vi "Begin[Conflict 1].vi"() -> (0 "Joystick 1 Error":errorcluster)   [LabVIEW 2013]
doc: "Called before other user functions, this VI is expected to open initial I/O refnums, load in file data, and do all program initialization. Notice that the <B>error out</B> terminal is simply used for data flow. Wiring it to other structures or subVIs ensures that this VI runs first."
uses:
  <vilib>/Rock Robotics/SystemInterfaces/DIO/FPGA_DIOPWMChannel.ctl
  <vilib>/Rock Robotics/WPI/SafetyOutput/WPI_SafetyOutputConfigMenu.ctl
  <vilib>/Rock Robotics/WPI/DriverStation/WPI_DriverStationRobotMode2.ctl
  <vilib>/Rock Robotics/SystemInterfaces/Typedef/FPGA_TypedefAnalogModuleForGyro.ctl
  <vilib>/Rock Robotics/SystemInterfaces/AI/FPGA_AIGyroChannel.ctl
  <vilib>/Rock Robotics/WPI/Joystick/WPI_JoystickDeviceEnum.ctl
  <vilib>/Rock Robotics/SystemInterfaces/DIO/FPGA_DIOChannel.ctl
  <vilib>/Rock Robotics/SystemInterfaces/DIO/FPGA_DIORelayChannel.ctl
  <vilib>/Rock Robotics/SystemInterfaces/Typedef/FPGA_TypedefSolenoidModule.ctl
  <vilib>/Rock Robotics/WPI/Solenoid/WPI_SolenoidChannel.ctl
  <vilib>/Rock Robotics/WPI/Solenoid/WPI_SolenoidValue.ctl
  <vilib>/Rock Robotics/WPI/RobotDrive/WPI_RobotDriveOpen2MotorWithTalon.vi
  Robot Global Data.vi
  <vilib>/Rock Robotics/WPI/Solenoid/WPI_SolenoidOpenDouble.vi
  <vilib>/Rock Robotics/WPI/Solenoid/WPI_SolenoidSetEnum.vi
  <vilib>/Rock Robotics/WPI/Solenoid/WPI_SolenoidOpenSingle.vi
  <vilib>/Rock Robotics/WPI/Compressor/WPI_CompressorGetSetRefNum.vi
panel:
  out "Motor Error":errorcluster
  out "Joystick 3 Error":errorcluster
  out "Gyro Open Error":errorcluster
  out "Joystick 2 Error":errorcluster
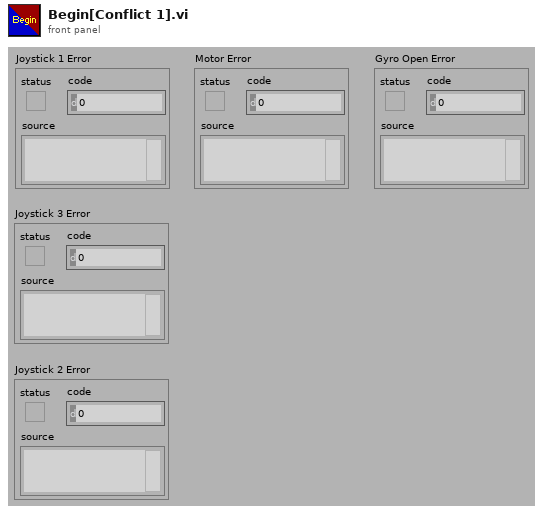
[diagram p1: front panel]
types:
  T1 = typedef "FPGA_DIORelayChannel.ctl" = enum8{"Relay 1", "Relay 2", "Relay 3", "Relay 4", "Relay 5", "Relay 6", "Relay 7", "Relay 8", "Invalid"}
  T2 = typedef "FPGA_DIOChannel.ctl" = enum8{"DIO 1", "DIO 2", "DIO 3", "DIO 4", "DIO 5", "DIO 6", "DIO 7", "DIO 8", "DIO 9", "DIO 10", "DIO 11", "DIO 12", "DIO 13", "DIO 14", "Invalid"}
  T3 = typedef "WPI_JoystickDeviceEnum.ctl" = enum16{"USB 1", "USB 2", "USB 3", "USB 4", "Kinect 1", "Kinect 2"}
  T4 = typedef "FPGA_AIGyroChannel.ctl" = enum8{"AI 1", "AI 2", "Invalid"}
  T5 = typedef "FPGA_TypedefAnalogModuleForGyro.ctl" = enum16{"Analog Module 1"}
  T6 = typedef "WPI_DriverStationRobotMode2.ctl" = enum16{"Autonomous Disabled", "Autonomous Enabled", "Teleop Disabled", "Teleop Enabled", "Timeout", "Finish", "Test Disabled", "Test Enabled"}
  T7 = typedef "WPI_SafetyOutputConfigMenu.ctl" = enum16{"Enable", "Disable"}
  T8 = typedef "FPGA_DIOPWMChannel.ctl" = enum8{"PWM 1", "PWM 2", "PWM 3", "PWM 4", "PWM 5", "PWM 6", "PWM 7", "PWM 8", "PWM 9", "PWM 10", "Invalid"}
  T9 = typedef "WPI_SolenoidChannel.ctl" = enum8{"Solenoid 1", "Solenoid 2", "Solenoid 3", "Solenoid 4", "Solenoid 5", "Solenoid 6", "Solenoid 7", "Solenoid 8", "Invalid"}
  T10 = typedef "FPGA_TypedefSolenoidModule.ctl" = enum16{"Solenoid Module 1", "Solenoid Module 2"}
  T11 = typedef "WPI_SolenoidDevRef.ctl" = cluster{"DevStatus":errorcluster, "Solenoid Module":T10, "Forward Solenoid Channel":T9, "Reverse Solenoid Channel":T9}
  T12 = typedef "WPI_SolenoidValue.ctl" = enum16{"Off", "On", "Forward", "Reverse"}
  T13 = typedef "WPI_JoystickDevRef.ctl" = cluster{"Device":T3}
  T14 = typedef "WPI_CompressorDevRef.ctl" = cluster{"DevStatus":errorcluster, "DigitalInputDevRef":T15, "RelayDevRef":T17}
  T15 = typedef "WPI_DigitalInputDevRef.ctl" = cluster{"DevStatus":errorcluster, "DIO Channel":T2, "Digital Module":T16}
  T16 = typedef "FPGA_TypedefDigitalModule.ctl" = enum16{"Digital Module 1", "Digital Module 2"}
  T17 = typedef "WPI_RelayDevRef.ctl" = cluster{"DevStatus":errorcluster, "Relay Channel":T1, "Digital Module":T16, "Relay Direction":T18}
  T18 = typedef "WPI_RelayDirection.ctl" = enum16{"Both directions", "Forward only", "Reverse only"}
  T19 = typedef "WPI_GyroDevRef.ctl" = cluster{"DevStatus":errorcluster, "Analog Module":T20, "Analog Channel":T21, "Offset":dbl, "Gain (VoltsPerDegree/Second)":dbl}
  T20 = typedef "FPGA_TypedefAnalogModule.ctl" = enum16{"Analog Module 1", "Analog Module 2"}
  T21 = typedef "FPGA_AIChannel.ctl" = enum8{"AI 1", "AI 2", "AI 3", "AI 4", "AI 5", "AI 6", "AI 7", "AI 8", "Invalid"}
  T22 = typedef "WPI_RobotDriveDevRef.ctl" = cluster{"DevStatus":errorcluster, "Motors[]":T23[], "Square Inputs":bool, "Max Output":dbl, "Isochronous":bool}
  T23 = typedef "WPI_MotorControlDeviceRef.ctl" = cluster{"DeviceStatus":errorcluster, "Type":enum16{"PWM", "CAN"}, "PWM":cluster{"Digital Module":T16, "PWM Channel":T8, "DeadBand":T24}, "CAN":cluster{"Device Number":u8, "Control Mode":T25, "Semaphore":T26, "Max Vout":dbl}, "Invert":bool, "TransformRef":T27, "InvTransformRef":T27}
  T24 = typedef "WPI_PWMDeadband.ctl" = cluster{"Name":string, "maxPositivePwm":i32, "minPositivePwm":i32, "centerPwm":i32, "maxNegativePwm":i32, "minNegativePwm":i32, "angularRange":u16}
  T25 = typedef "WPI_CANJaguar_ControlMode.ctl" = enum8{"Percent VBus", "Current", "Speed", "Position", "Voltage"}
  T26 = typedef "Semaphore RefNum" = refnum<k1>
  T27 = typedef "WPI_PWMTransform_ConPane.ctl" = refnum<vi>
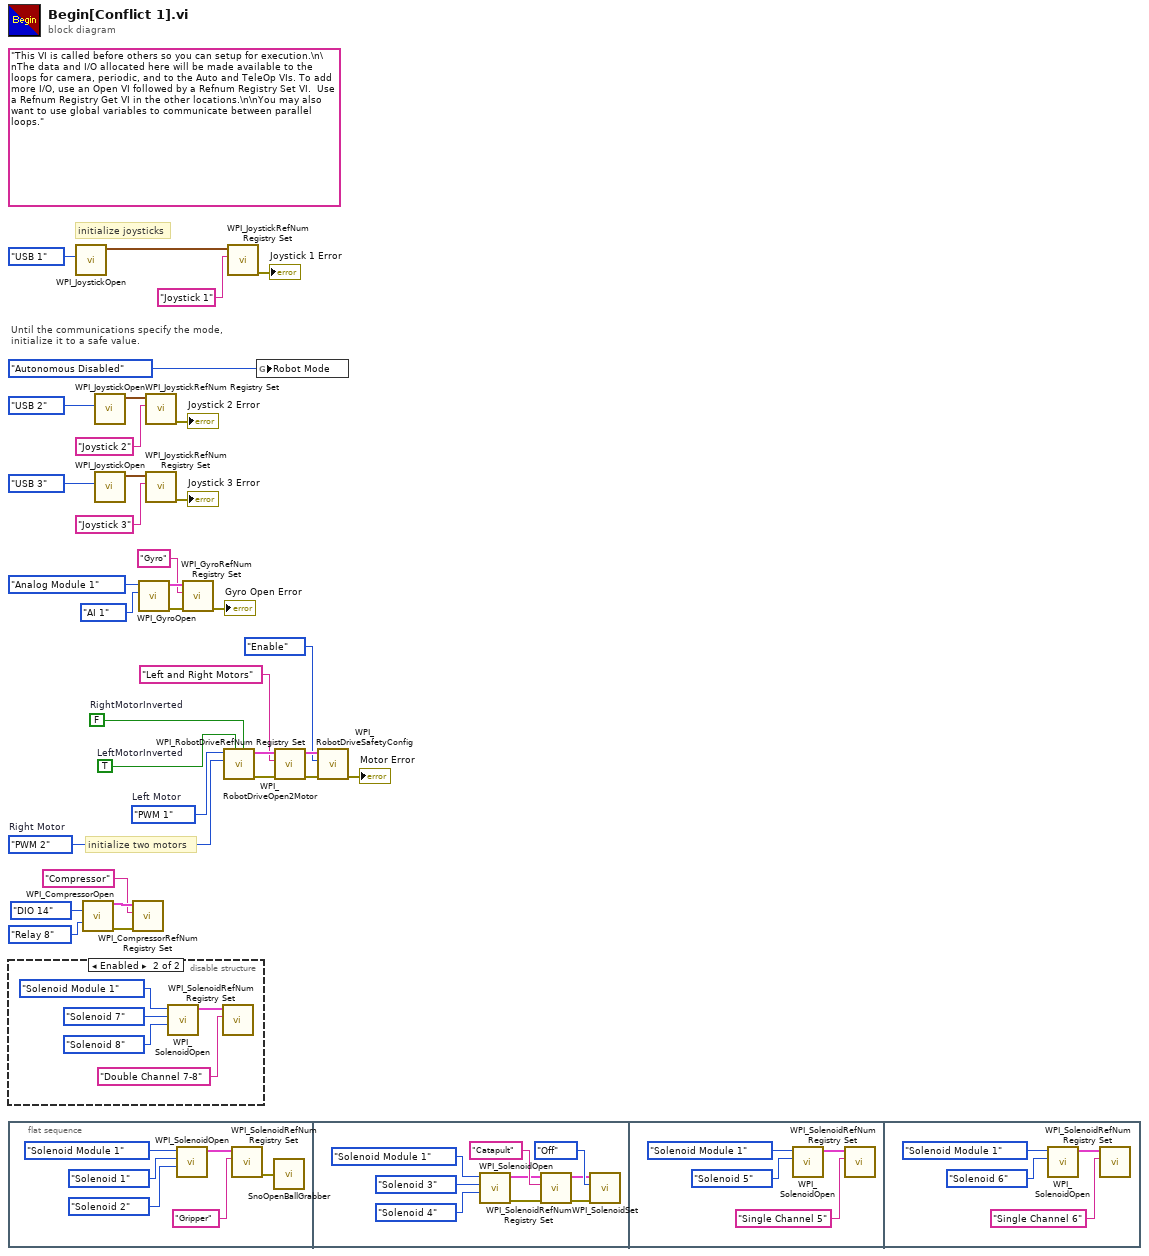
[diagram p0: block diagram]
diagram:
  (unwired) "This VI is called before others so you can setup for execution.\n\nThe data and I/O allocated here will be made available to the loops for camera, periodic, and to the Auto and TeleOp VIs. To add more I/O, use an Open VI followed by a Refnum Registry Set VI.  Use a Refnum Registry Get VI in the other locations.\n\nYou may also want to use global variables to communicate between parallel loops."
  w29 = FPGA_DIOPWMChannel."PWM 2"  # Right Motor
  w30 = FPGA_DIOPWMChannel."PWM 1"  # Left Motor
  w34 = TRUE  # LeftMotorInverted
  w35 = FALSE  # RightMotorInverted
  # "initialize joysticks"
  # "Until the communications specify the mode,\ninitialize it to a safe value."
  # "initialize two motors"
  n1 = disable-structure shown="Enabled" {
    frame Disabled {
    }
    frame Enabled {
      n2 = call-poly <vilib>:"WPI_SolenoidOpen.vi"("Reverse Solenoid Channel"=WPI_SolenoidChannel."Solenoid 8", "Forward Solenoid Channel"=WPI_SolenoidChannel."Solenoid 7", "Solenoid Module (Module 1)"=FPGA_TypedefSolenoidModule."Solenoid Module 1") -> ("SolenoidDevRef"=w39:T11)  [unwired: 7 in, 1 out]
      n3 = call <vilib>:"WPI_SolenoidRefNum Registry Set.vi"("refnum name"="Double Channel 7-8", "SolenoidDevRef"=w39) -> ()  [unwired: 8 in, 2 out]
    }
  }
  n4 = flat-sequence {
    frame #0 {
      n5 = call-poly <vilib>:"WPI_SolenoidOpen.vi"("Reverse Solenoid Channel"=WPI_SolenoidChannel."Solenoid 2", "Forward Solenoid Channel"=WPI_SolenoidChannel."Solenoid 1", "Solenoid Module (Module 1)"=FPGA_TypedefSolenoidModule."Solenoid Module 1") -> ("SolenoidDevRef"=w46:T11)  [unwired: 7 in, 1 out]
      n6 = call <vilib>:"WPI_SolenoidRefNum Registry Set.vi"("refnum name"="Gripper", "SolenoidDevRef"=w46) -> ("error out"=w41:errorcluster)  [unwired: 8 in, 1 out]
      n7 = call "SnoOpenBallGrabber.vi"("Input Error"=w41) -> ()  [unwired: 1 out]
    }
    frame #1 {
      n8 = call-poly <vilib>:"WPI_SolenoidOpen.vi"("Reverse Solenoid Channel"=WPI_SolenoidChannel."Solenoid 4", "Forward Solenoid Channel"=WPI_SolenoidChannel."Solenoid 3", "Solenoid Module (Module 1)"=FPGA_TypedefSolenoidModule."Solenoid Module 1") -> ("error out"=w51:errorcluster, "SolenoidDevRef"=w50:T11)  [unwired: 7 in]
      n9 = call <vilib>:"WPI_SolenoidRefNum Registry Set.vi"("error in (no error)"=w51, "refnum name"="Catapult", "SolenoidDevRef"=w50) -> ("error out"=w54:errorcluster, "SolenoidDevRef"=w53:T11)  [unwired: 7 in]
      n10 = call-poly <vilib>:"WPI_SolenoidSet.vi"("error in (no error)"=w54, "Value"=WPI_SolenoidValue."Off", "SolenoidDevRef"=w53) -> ()  [unwired: 7 in, 2 out]
    }
    frame #2 {
      n11 = call-poly <vilib>:"WPI_SolenoidOpen.vi"("Solenoid Channel"=WPI_SolenoidChannel."Solenoid 5" ("Forward Solenoid Channel"), "Solenoid Module (Module 1)"=FPGA_TypedefSolenoidModule."Solenoid Module 1") -> ("SolenoidDevRef"=w58:T11)  [unwired: 8 in, 1 out]
      n12 = call <vilib>:"WPI_SolenoidRefNum Registry Set.vi"("refnum name"="Single Channel 5", "SolenoidDevRef"=w58) -> ()  [unwired: 8 in, 2 out]
    }
    frame #3 {
      n13 = call-poly <vilib>:"WPI_SolenoidOpen.vi"("Solenoid Channel"=WPI_SolenoidChannel."Solenoid 6" ("Forward Solenoid Channel"), "Solenoid Module (Module 1)"=FPGA_TypedefSolenoidModule."Solenoid Module 1") -> ("SolenoidDevRef"=w62:T11)  [unwired: 8 in, 1 out]
      n14 = call <vilib>:"WPI_SolenoidRefNum Registry Set.vi"("refnum name"="Single Channel 6", "SolenoidDevRef"=w62) -> ()  [unwired: 8 in, 2 out]
    }
  }
  n15 = call <vilib>:"WPI_JoystickOpen.vi"("JoystickDevice"=WPI_JoystickDeviceEnum."USB 1") -> ("JoystickDevRef"=w13:T13)  [unwired: 10 in]
  n16 = call <vilib>:"WPI_CompressorOpen.vi"("Pressure Switch DIO Channel"=FPGA_DIOChannel."DIO 14", "Relay Channel"=FPGA_DIORelayChannel."Relay 8") -> ("CompressorDevRef"=w3:T14, "error out"=w2:errorcluster)  [unwired: 12 in]
  n17 = call <vilib>:"WPI_JoystickOpen.vi"("JoystickDevice"=WPI_JoystickDeviceEnum."USB 2") -> ("JoystickDevRef"=w17:T13)  [unwired: 10 in]
  n18 = call <vilib>:"WPI_JoystickOpen.vi"("JoystickDevice"=WPI_JoystickDeviceEnum."USB 3") -> ("JoystickDevRef"=w9:T13)  [unwired: 10 in]
  n19 = call <vilib>:"WPI_CompressorRefNum Registry Set.vi"("error in (no error)"=w2, "refnum name"="Compressor", "CompressorDevRef"=w3) -> ()  [unwired: 7 in, 2 out]
  n20 = call <vilib>:"WPI_GyroOpen.vi"("Analog Channel"=FPGA_AIGyroChannel."AI 1", "Analog Module (Module 1)"=FPGA_TypedefAnalogModuleForGyro."Analog Module 1") -> ("error out"=w21:errorcluster, "GyroDevRef"=w23:T19)  [unwired: 7 in, 1 out]
  n21 = call <vilib>:"WPI_JoystickRefNum Registry Set.vi"("refnum name"="Joystick 2", "JoystickDevRef"=w17) -> ("error out"=→"Joystick 2 Error":errorcluster)  [unwired: 8 in, 1 out]
  n22 = call <vilib>:"WPI_JoystickRefNum Registry Set.vi"("refnum name"="Joystick 3", "JoystickDevRef"=w9) -> ("error out"=→"Joystick 3 Error":errorcluster)  [unwired: 8 in, 1 out]
  n23 = call <vilib>:"WPI_GyroRefNum Registry Set.vi"("error in (no error)"=w21, "refnum name"="Gyro", "GyroDevRef"=w23) -> ("error out"=→"Gyro Open Error":errorcluster)  [unwired: 7 in, 1 out]
  n24 = call-poly <vilib>:"WPI_RobotDriveOpen2Motor.vi"("Right Motor Inverted"=w35, "Left Motor Inverted"=w34, "Right Motor"=w29, "Left Motor"=w30) -> ("error out"=w31:errorcluster, "RobotDriveDevRef"=w33:T22)  [unwired: 1 in, 5 out]
  n25 = call <vilib>:"WPI_JoystickRefNum Registry Set.vi"("refnum name"="Joystick 1", "JoystickDevRef"=w13) -> ("error out"=→"Joystick 1 Error":errorcluster)  [unwired: 8 in, 1 out]
  n26 = global write "Robot Global Data.vi" "Robot Mode"(WPI_DriverStationRobotMode2."Autonomous Disabled" ("Robot Mode")) -> ()
  n27 = call <vilib>:"WPI_RobotDriveRefNum Registry Set.vi"("error in (no error)"=w31, "refnum name"="Left and Right Motors", "RobotDriveDevRef"=w33) -> ("error out"=w7:errorcluster, "RobotDriveDevRef"=w28:T22)  [unwired: 7 out]
  n28 = call <vilib>:"WPI_RobotDriveSafetyConfig.vi"("error in (no error)"=w7, "mode"=WPI_SafetyOutputConfigMenu."Enable", "RobotDriveDevRef"=w28) -> ("error out"=→"Motor Error":errorcluster)  [unwired: 7 in, 1 out]
